vi "CVT2NoTagsTest.vi"() -> (3 "Unit Test Framework Results":T1)   [LabVIEW 2013, in "UnitTests.lvlib"]
uses:
  UnitTests.lvlib
  <vilib>/utf/common/utf_test_result_troll.ctl
  <vilib>/utf/common/utf_test_result.ctl
  <vilib>/utf/common/utf_test_result_failure.ctl
  <vilib>/utf/common/utf_test_comparison_operators.ctl
  <vilib>/utf/common/utf_vi_tag.ctl
  <vilib>/NI/Current Value Table/Type Defs/File Format.ctl
  <vilib>/NI/Current Value Table/Type Defs/Single Tag.ctl
  <vilib>/NI/Current Value Table/Type Defs/Data Types.ctl
  <vilib>/NI/Current Value Table/Type Defs/Tag Grouping set.ctl
  <vilib>/utf/NI_UnitTestFramework.lvlib
  <vilib>/NI/Current Value Table/Current Value Table.lvlib
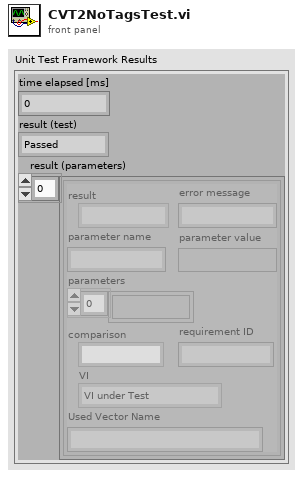
[diagram p1: front panel]
types:
  T1 = typedef "NI_UnitTestFramework.lvlib/utf_test_result_troll.ctl" = cluster{"time elapsed [ms]":u32, "result (test)":T2, "result (parameters)":T3[]}
  T2 = typedef "NI_UnitTestFramework.lvlib/utf_test_result.ctl" = enum16{"Passed", "Failed", "Error", "Skipped", "Not Processed"}
  T3 = typedef "NI_UnitTestFramework.lvlib/utf_test_result_failure.ctl" = cluster{"result":T2, "error message":string, "parameter name":string, "parameter value":variant, "parameters":variant[], "comparison":T4, "requirement ID":string, "VI":T5, "Used Vector Name":string}
  T4 = typedef "NI_UnitTestFramework.lvlib/utf_test_comparison_operators.ctl" = enum16{"=", "!=", ">", ">=", "<", "<=", "range", "symmetric tolerance", "asymmetric tolerance", "string contains", "string not contain", "array size", "string length", "array range", "by element", "array range (limit array)", "user-defined", "array contains", "array not contain", "vector length", "= (elm)", "!= (elm)", "= (case insensitive)", "!= (case insensitive)"}
  T5 = typedef "NI_UnitTestFramework.lvlib/utf_vi_tag.ctl" = enum16{"Setup VI", "VI under Test", "Teardown VI"}
  T6 = typedef "Current Value Table.lvlib/File Format.ctl" = cluster{"Tags":T7[], "Group Listings":T9[]}
  T7 = typedef "Current Value Table.lvlib/Single Tag.ctl" = cluster{"Data Type":T8, "Name":string, "Value":string, "Description":string}
  T8 = typedef "Current Value Table.lvlib/Data Types.ctl" = enum16{"Double", "Single", "I64", "I32", "I16", "I8", "U64", "U32", "U16", "U8", "String", "Boolean", "Array of U8", "Array of U16", "Array of U32", "Array of U64", "Array of I64", "Array of I32", "Array of I16", "Array of I8", "Array of Double", "Array of Single", "Array of Boolean", "Array of String"}
  T9 = typedef "Current Value Table.lvlib/Tag Grouping set.ctl" = cluster{"Group":string, "Tag Names":string[]}
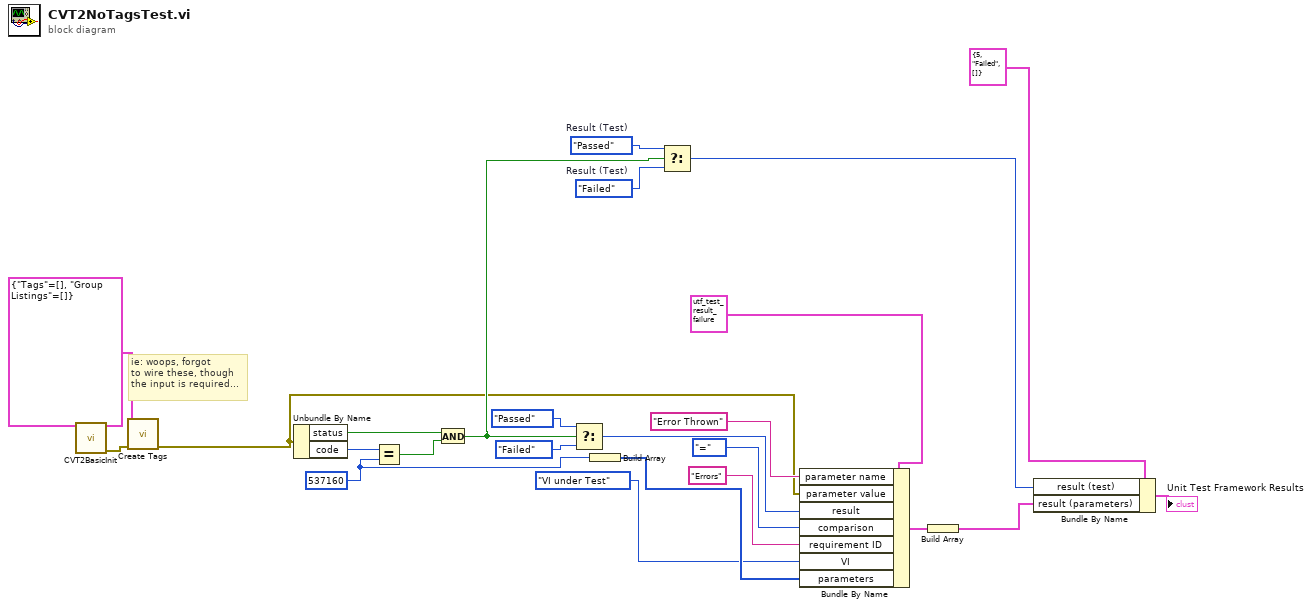
[diagram p0: block diagram]
diagram:
  w15 = utf_test_result."Passed"  # Result (Test)
  w16 = utf_test_result."Failed"  # Result (Test)
  w10 = 537160 ("y")
  # "ie: woops, forgot\nto wire these, though\nthe input is required..."
  n1 = call "CVT2BasicInit.vi"() -> ("error out"=w3:errorcluster)  [unwired: 9 in, 2 out]
  n2 = call <vilib>:"Create Tags.vi"("error in (no error)"=w3, "CVT Tags to Create"=T6 {"Tags"=[], "Group Listings"=[]} ("CVT Tags to Load")) -> ("error out"=w2:errorcluster)  [unwired: 9 in]
  n3 = Unbundle By Name(w2) -> ("status"=w4:bool, "code"=w5:i32)
  n4 = Equal?(x=w5, y=w10) -> (x = y?=w19:bool)
  n5 = And(x=w4, y=w19) -> (x .and. y?=w6:bool)
  n6 = Select(t=utf_test_result."Passed" ("result"), s=w6, f=utf_test_result."Failed" ("result")) -> (s? t:f=w12:T2)
  n7 = Build Array(w10) -> (w11:i32[])
  n8 = Select(t=w15, s=w6, f=w16) -> (s? t:f=w14:T2)
  n9 = Bundle By Name(cluster=T3 {"result"=enum."Passed", "error message"="", "parameter name"="", "parameter value"=variant, "parameters"=[], "comparison"=enum."=", "requirement ID"="", "VI"=enum."Setup VI", "Used Vector Name"=""} ("Unit Test Framework - result (parameters)"), "parameter name"="Error Thrown", "parameter value"=w2, "result"=w12, "comparison"=utf_test_comparison_operators."=", "requirement ID"="Errors" ("parameter name"), "VI"=utf_vi_tag."VI under Test", "parameters"=w11) -> (w21:T3)
  n10 = Build Array(w21) -> (w13:T3[])
  n11 = Bundle By Name(cluster=T1 {"time elapsed [ms]"=5, "result (test)"=enum."Failed", "result (parameters)"=[]} ("Unit Test Framework - Result"), "result (test)"=w14, "result (parameters)"=w13) -> (→"Unit Test Framework Results":T1)
